vi "FTW-Endpoint-TCP-Multipart-Ask.vi"(0 "FTW Endpoint":refnum<class "FTW-Endpoint-TCP.lvclass">, 5 "Multipart Message":string[](array[string]), 7 "Read Timeout":i32=1000 format="%dmsec", 9 "Write Timeout":i32=-1 format="%dmsec", 11 "error in":errorcluster) -> (4 "FTW Endpoint out":refnum<class "FTW-Endpoint-TCP.lvclass">, 6 "Reply":string[](array[string]), 8 "Read Timed out?":bool, 10 "Write Timed out?":bool, 15 "error out":errorcluster)   [LabVIEW 2013, in "FTW-Endpoint-TCP.lvclass"]
uses:
  FTW-Endpoint-TCP.lvclass
  Ether/FTW-Ether.lvclass
panel:
  # "Inputs"
  # "Outputs"
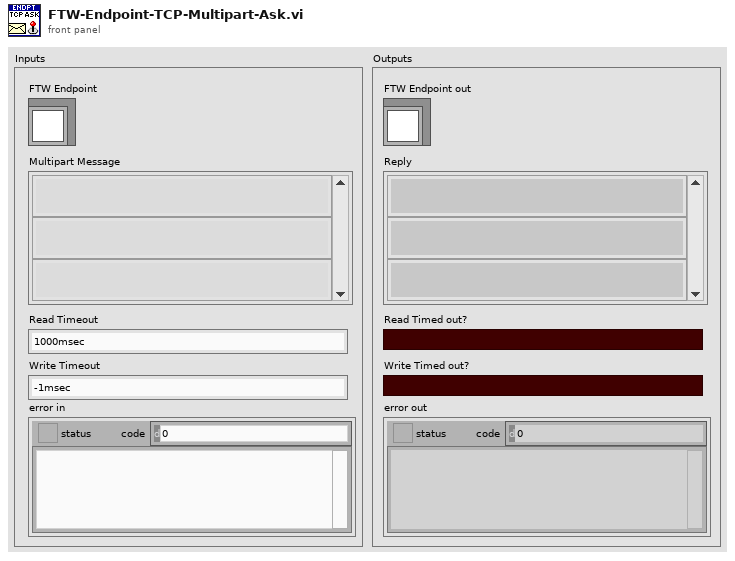
[diagram p1: front panel]
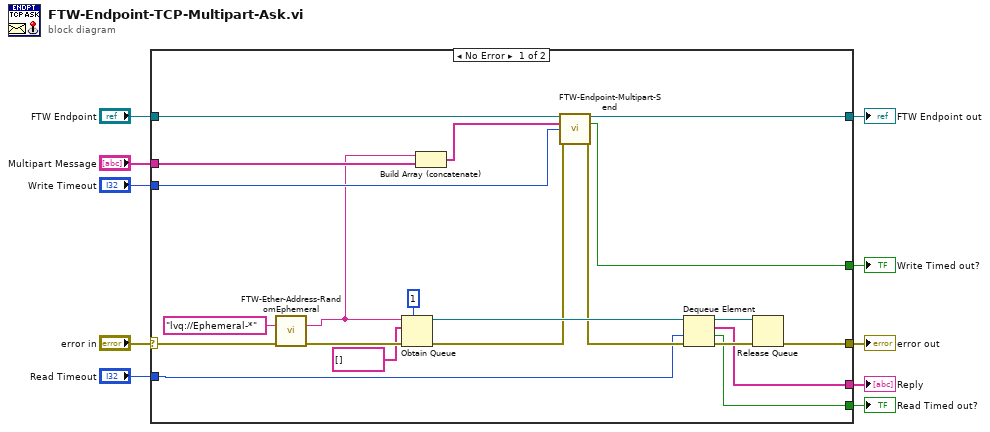
[diagram p0: block diagram]
diagram:
  n1 = case shown="No Error" "error in" {
    selector: "error in" -> [w21 w33]
    tunnel: [w12 w33] -> w10
    tunnel: [w17 w32] -> w8
    tunnel: "FTW Endpoint" -> [w29 w32]
    tunnel: "Multipart Message" -> [w31 _]
    tunnel: "Read Timeout" -> [w15 _]
    tunnel: "Write Timeout" -> [w30 _]
    tunnel: [w14 _] -> w3
    tunnel: [w13 _] -> w2
    tunnel: [w11 _] -> w1
    frame No Error {
      n2 = call "FTW-Ether-Address-RandomEphemeral.vi"("Endpoint"="lvq://Ephemeral-*" ("Requested Ephemeral Address"), "error in"=w21) -> ("Endpoint with Replacements"=w20:string, "error out"=w25:errorcluster)  [unwired: 12 in]
      n3 = Obtain Queue(max queue size (-1, unlimited)=1, name (unnamed)=w20, element data type=string[] [], error in (no error)=w25) -> (queue out=w22:refnum<queue>, error out=w18:errorcluster)  [unwired: 1 in, 1 out]
      n4 = Build Array (concatenate)(w20, w31) -> (w19:string[])
      n5 = call-dynamic "FTW-Endpoint-Multipart-Send.vi"("FTW Endpoint"=w29, "Multipart Message"=w19, "Timeout"=w30, "error in"=w18) -> ("FTW Endpoint out"=w17:refnum<class "FTW-Endpoint-TCP.lvclass">, "Timed out?"=w11:bool, "error out"=w16:errorcluster)  [unwired: 9 in]
      n6 = Dequeue Element(queue=w22, timeout in ms (-1)=w15, error in (no error)=w16) -> (queue out=w28:refnum<queue>, element=w14:string[], timed out?=w13:bool, error out=w27:errorcluster)
      n7 = Release Queue(queue=w28, error in (no error)=w27) -> (error out=w12:errorcluster)  [unwired: 1 in, 2 out]
    }
    frame Error {
    }
  }
  "error out" <- w10
  "FTW Endpoint out" <- w8
  "Read Timed out?" <- w2
  "Reply" <- w3
  "Write Timed out?" <- w1
